vi "4 channels no handoff 2024.vi"() -> ()   [LabVIEW 2022 SP3]
uses:
  <vilib>/DAQmx/write.llb/DAQmx Write (Digital 1D Bool NChan 1Samp 1Line).vi
  <vilib>/DAQmx/create/channels.llb/DAQmx Create Channel (DI-Digital Input).vi
  <vilib>/DAQmx/miscellaneous.llb/DAQmx Fill In Error Info.vi
panel:
  out "error out":errorcluster
  in  "lines":tag
  out "Blue":bool
  in  "Loop Time (ms)":u32=50
  in  "U":bool
  out "Yellow":bool
  out "Orange":bool
  out "Pink":bool
  in  "stop":bool
  # "TO RIGHT"
  # "TO LEFT"
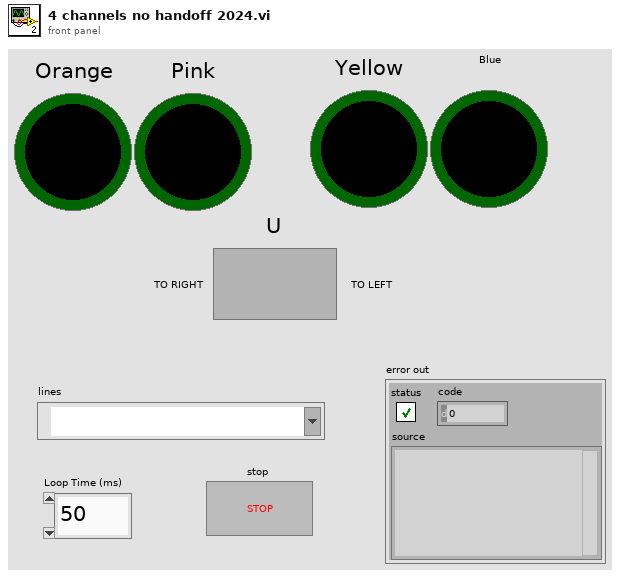
[diagram p1: front panel]
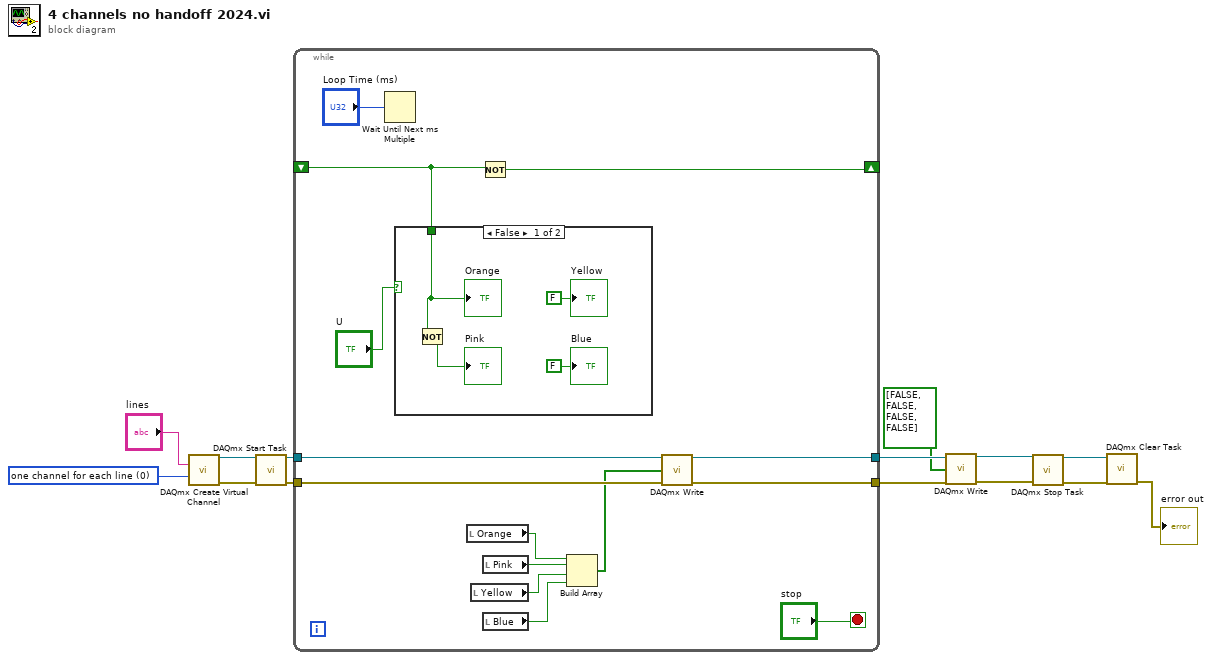
[diagram p0: block diagram]
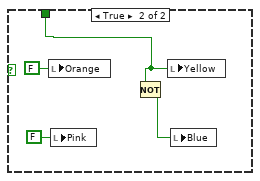
[diagram p2: hidden frame]
diagram:
  w13 = 0 items=["one channel for each line", "one channel for all lines"] ("line grouping")
  n1 = call-poly <vilib>:"DAQmx Create Virtual Channel.vi"("lines"="lines", "line grouping"=w13) -> ("task out"=w12:refnum<k21>, "error out"=w11:errorcluster)  [unwired: 12 in]
  n2 = call <vilib>:"DAQmx Start Task.vi"("task/channels in"=w12, "error in"=w11) -> ("task out"=w10:refnum<k21>, "error out"=w9:errorcluster)  [unwired: 12 in]
  n3 = while {
    shift-right: [w27] -> _
    shift-left: _ -> [w25]
    tunnel: w10 -> [w19]
    tunnel: w9 -> [w18]
    tunnel: [w16] -> w8
    tunnel: [w15] -> w7
    stop <- "stop" stop-if-true
    n4 = Wait Until Next ms Multiple(millisecond multiple="Loop Time (ms)") -> ()  [unwired: 1 out]
    n5 = case shown="False" "U" {
      tunnel: w25 -> [w30 w36]
      frame False {
        n6 = Not(x=w30) -> (.not. x?=→"Pink":bool)
        "Orange" <- w30
        "Yellow" <- FALSE ("Yellow")
        "Blue" <- FALSE ("Blue")
      }
      frame True {
        n7 = local write "Orange"(FALSE ("Orange")) -> ()
        n8 = local write "Pink"(FALSE ("Pink")) -> ()
        n9 = Not(x=w36) -> (.not. x?=w33:bool)
        n10 = local write "Yellow"(w36) -> ()
        n11 = local write "Blue"(w33) -> ()
      }
    }
    n12 = local read "Orange"() -> (w24:bool)
    n13 = local read "Yellow"() -> (w22:bool)
    n14 = Not(x=w25) -> (.not. x?=w27:bool)
    n15 = local read "Pink"() -> (w23:bool)
    n16 = local read "Blue"() -> (w21:bool)
    n17 = Build Array(w24, w23, w22, w21) -> (w17:bool[])
    n18 = call-poly <vilib>:"DAQmx Write.vi"("task/channels in"=w19, "data"=w17, "error in"=w18) -> ("task out"=w16:refnum<k21>, "error out"=w15:errorcluster)  [unwired: 10 in, 1 out]
  }
  n19 = call-poly <vilib>:"DAQmx Write.vi"("task/channels in"=w8, "data"=bool[] [FALSE, FALSE, FALSE, FALSE], "error in"=w7) -> ("task out"=w6:refnum<k21>, "error out"=w5:errorcluster)  [unwired: 10 in, 1 out]
  n20 = call <vilib>:"DAQmx Stop Task.vi"("task/channels in"=w6, "error in"=w5) -> ("task out"=w3:refnum<k21>, "error out"=w2:errorcluster)  [unwired: 12 in]
  n21 = call <vilib>:"DAQmx Clear Task.vi"("task in"=w3, "error in"=w2) -> ("error out"=→"error out":errorcluster)  [unwired: 13 in]
